vi "sub split frame string.vi"(8 "error in (no error)":errorcluster, 11 "frame string":string="<f 23 -\n   pic 73 state 3 wait 1 next 999 centerx 33\n   <bp x 56.320136999999995 y 45.18847 bp>\n   <w kind 1 x 65.42343 y 62.40722 weaponact 24 w>\n   <b kind 0 x 23 y 14 w 36 h 66 b>\n   <b kind 0 x 30 y 66 w 17 h 18 b>\nf>") -> (0 "error out":errorcluster, 3 "split string":T1)   [LabVIEW 2018, in "Frame Analizer.lvclass"]
uses:
  Frame Analizer.lvclass
panel:
  out "debug first subarray":string[](array[string])
  out "debug array":string[](array[string])
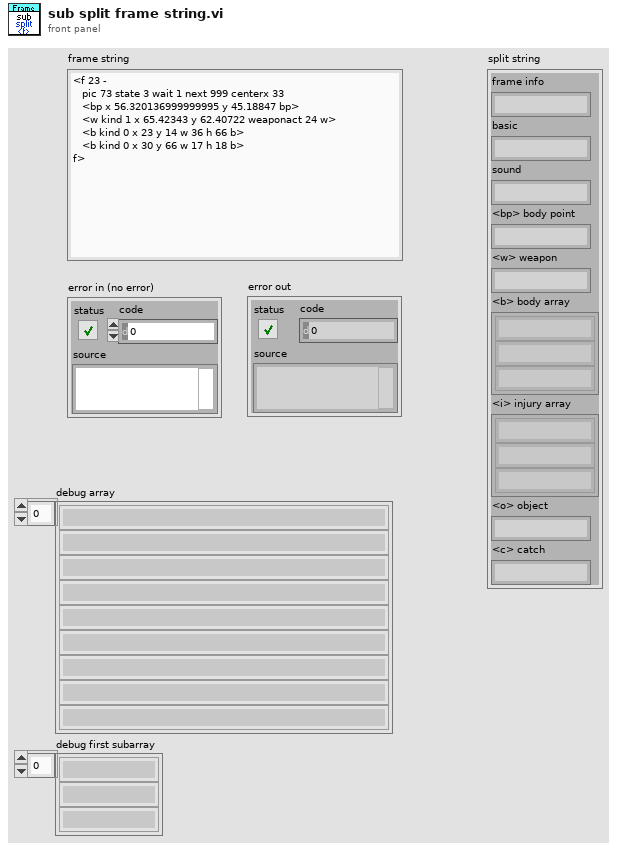
[diagram p1: front panel]
types:
  T1 = cluster{"frame info":string, "basic":string, "sound":string, "<bp> body point":string, "<w> weapon":string, "<b> body array":string[], "<i> injury array":string[], "<o> object":string, "<c> catch":string}
  T2 = cluster{string, string, "String":string, "String":string, "String":string, "filted string array":string[], "filted string array":string[], "String":string, "String":string}
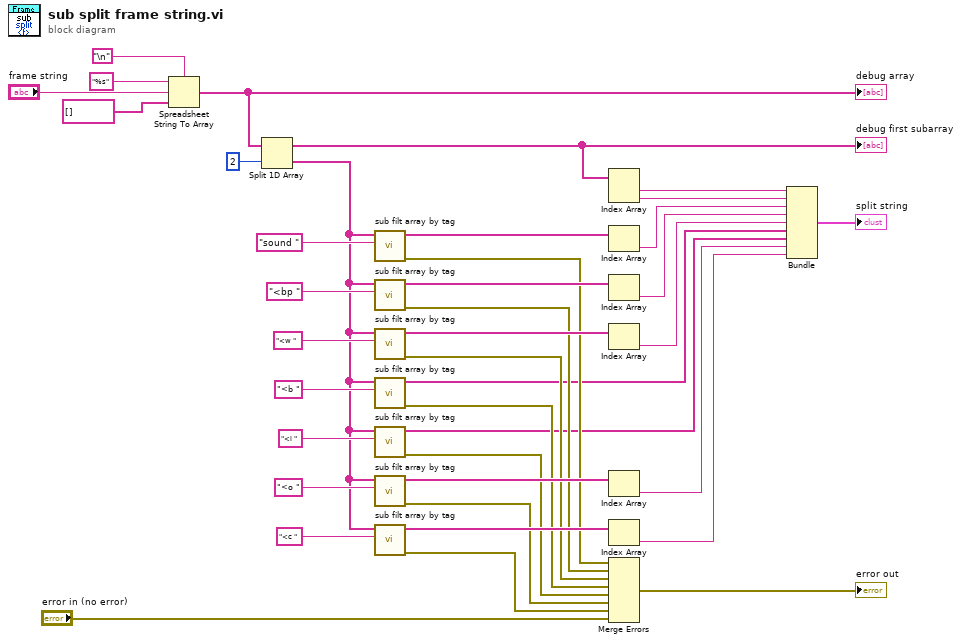
[diagram p0: block diagram]
diagram:
  n1 = Spreadsheet String To Array(delimiter (Tab)="\n", format string="%s", spreadsheet string="frame string", array type (2D Dbl)=string[] []) -> (array=w35:string[])
  "debug array" <- w35
  n2 = Split 1D Array(array=w35, index=2) -> (first subarray=w13:string[], second subarray=w21:string[])
  "debug first subarray" <- w13
  n3 = call "sub filt array by tag.vi"("tag"="sound ", "string array"=w21) -> ("error out"=w20:errorcluster, "filted string array"=w32:string[])  [unwired: 8 in]
  n4 = call "sub filt array by tag.vi"("tag"="<bp ", "string array"=w21) -> ("error out"=w19:errorcluster, "filted string array"=w31:string[])  [unwired: 8 in]
  n5 = call "sub filt array by tag.vi"("tag"="<w ", "string array"=w21) -> ("error out"=w18:errorcluster, "filted string array"=w30:string[])  [unwired: 8 in]
  n6 = call "sub filt array by tag.vi"("tag"="<b ", "string array"=w21) -> ("error out"=w17:errorcluster, "filted string array"=w7:string[])  [unwired: 8 in]
  n7 = call "sub filt array by tag.vi"("tag"="<i ", "string array"=w21) -> ("error out"=w16:errorcluster, "filted string array"=w1:string[])  [unwired: 8 in]
  n8 = call "sub filt array by tag.vi"("tag"="<o ", "string array"=w21) -> ("error out"=w15:errorcluster, "filted string array"=w29:string[])  [unwired: 8 in]
  n9 = call "sub filt array by tag.vi"("tag"="<c ", "string array"=w21) -> ("error out"=w14:errorcluster, "filted string array"=w23:string[])  [unwired: 8 in]
  n10 = Index Array(array=w13) -> (element #1=w12:string, element #2=w11:string)  [unwired: 2 in]
  n11 = Index Array(array=w32) -> (element=w10:string)  [unwired: 1 in]
  n12 = Index Array(array=w31) -> (element=w9:string)  [unwired: 1 in]
  n13 = Index Array(array=w30) -> (element=w8:string)  [unwired: 1 in]
  n14 = Index Array(array=w29) -> (element=w6:string)  [unwired: 1 in]
  n15 = Index Array(array=w23) -> (element=w5:string)  [unwired: 1 in]
  n16 = Merge Errors(w20, w19, w18, w17, w16, w15, w14, "error in (no error)") -> (→"error out":errorcluster)
  n17 = Bundle(w12, w11, "String"=w10, "String"=w9, "String"=w8, "filted string array"=w7, "filted string array"=w1, "String"=w6, "String"=w5) -> (→"split string":T2)  [unwired: 1 in]
